vi "Logger2_Loop.vi"(8 "error in (no error)":errorcluster) -> (0 "error out":errorcluster)   [LabVIEW 2016]
uses:
  Classes/DataLogger/Data Logger.lvclass
  <vilib>/Platform/TimedLoop/XDataNode/timing_clust.ctl
  <vilib>/Platform/TimedLoop/XDataNode/nitl_modes.ctl
  <vilib>/Platform/TimedLoop/XDataNode/wakeup.ctl
  <vilib>/Platform/TimedLoop/XDataNode/XDataNode.xnode
  <vilib>/Platform/TimedLoop/XDataNode/XDNodeRunTimeDep.lvlib
  <vilib>/GoldZinc Software/auzn custom VIs/CustomVI.lvlib
panel:
  out "Save Time":dbl
  out "ColumnOfVar":i32[](array[numeric])
  out "NumOfColumn":i32
  out "StartTime":dbl
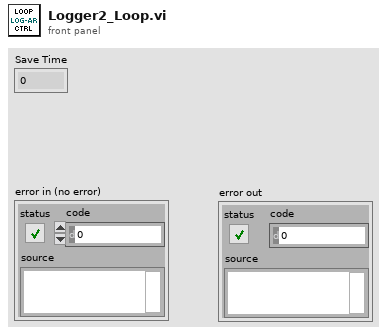
[diagram p1: front panel]
types:
  T1 = enum16{"Idle", "CloseFile", "WriteFile", "CreateFile"}
  T2 = typedef "XDNodeRunTimeDep.lvlib/timing_clust.ctl" = cluster{"Expected End [f-1]":u64, "Actual End [f-1]":u64, "Finished Late? [f-1]":bool, "Expected End [i-1]":u64, "Actual End [i-1]":u64, "Finished Late? [i-1]":bool, "Expected Start [i]":u64, "Actual Start [i]":u64, "Expected Start [f]":u64, "Actual Start [f]":u64, "Source Name":string, "Structure Name":string, "Period":i64, "Deadline":i64, "Offset":i64, "Start":i64, "Priority":i32, "Timeout":i32, "Mode":T3, "Wakeup Reason":T4, "Error":errorcluster, "Source Type":string, "Secondary Source Type":string, "Global End Time":u64, "Global Start Time":u64, "Frame Duration":u64, "Iteration Duration":u64, "Assigned CPU":i32, "I/O Scan Engine Mode":u32}
  T3 = typedef "XDNodeRunTimeDep.lvlib/nitl_modes.ctl" = enum32{"No Change", "Process missed periods, maintain original phase", "Discard missed periods, maintain original phase", "Process missed periods, ignore original phase", "Discard missed periods, ignore original phase"}
  T4 = typedef "XDNodeRunTimeDep.lvlib/wakeup.ctl" = enum32{"Normal", "Aborted", "Asynchronous wakeup", "Timing source error", "Timed loop error", "Timeout"}
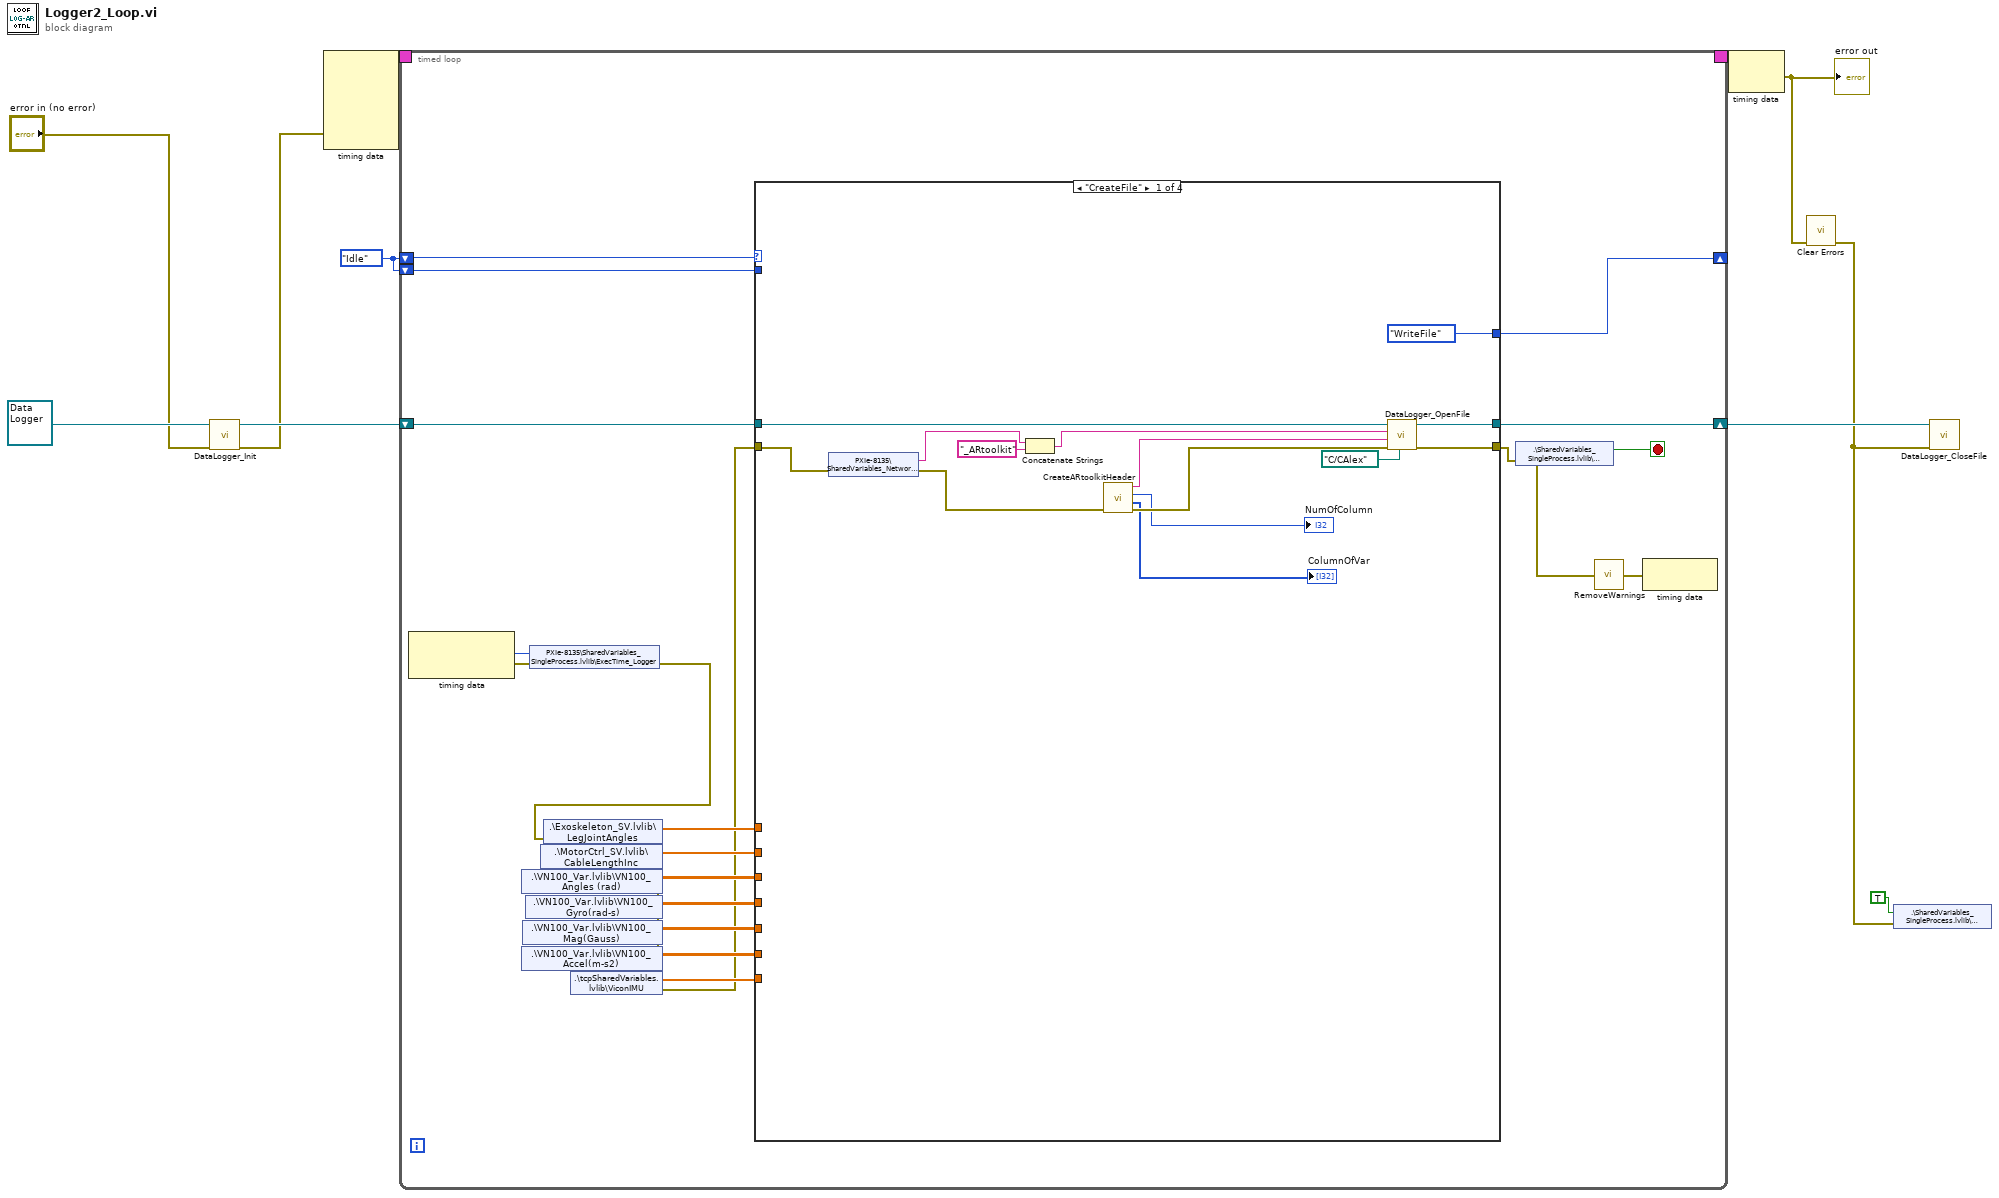
[diagram p0: block diagram]
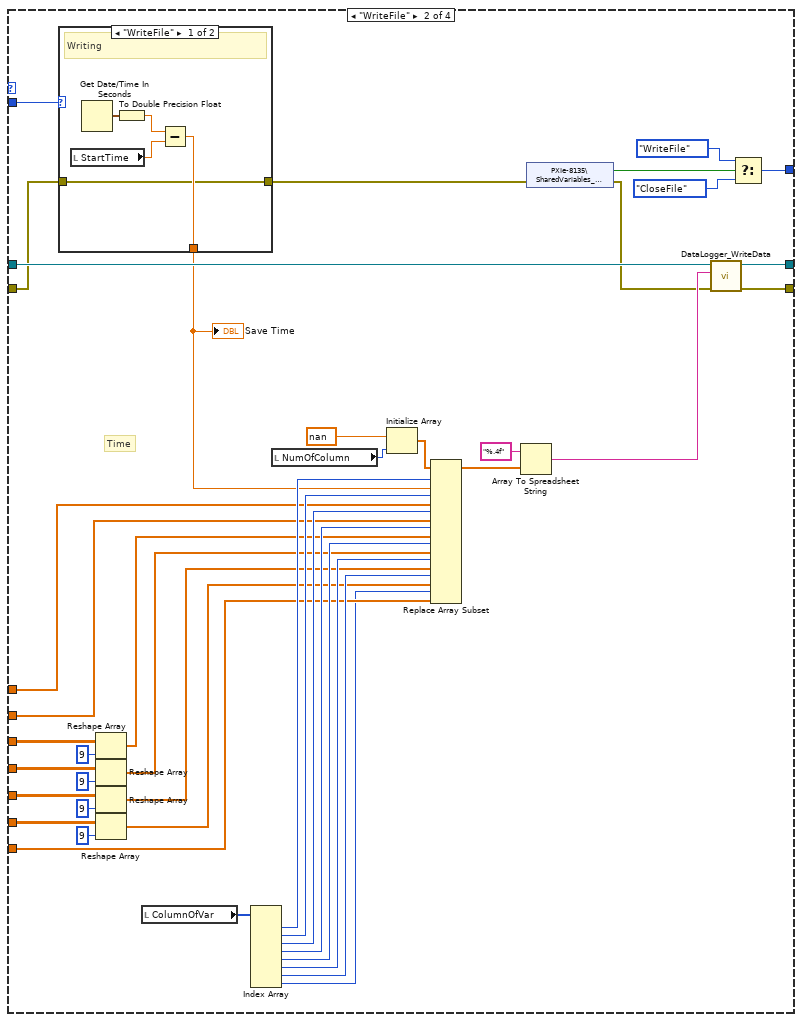
[diagram p2: hidden frame]
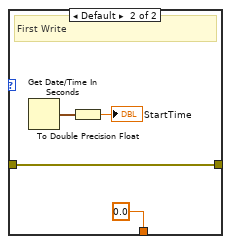
[diagram p3: hidden frame]
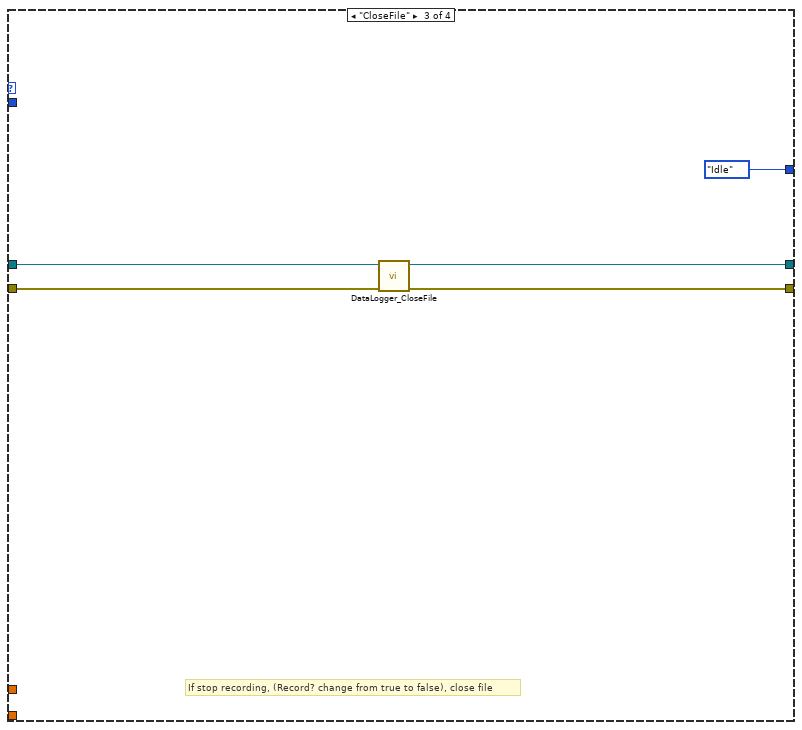
[diagram p4: hidden frame]
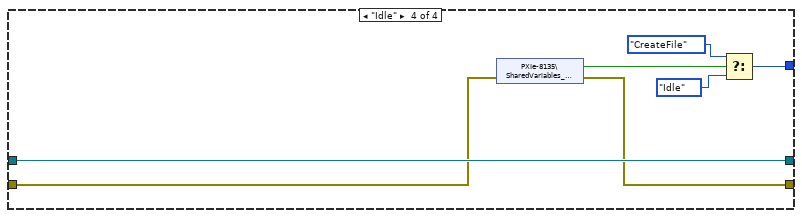
[diagram p5: hidden frame]
diagram:
  w9 = T1."Idle"
  n1 = call "DataLogger_Init.vi"("error in (no error)"="error in (no error)", "Data Logger in"=refnum<class "Data Logger.lvclass"> refnum) -> ("error out"=w1:errorcluster, "Data Logger out"=w3:refnum<class "Data Logger.lvclass">)  [unwired: 8 in]
  n2 = node-c288(w1) -> (w11:T2)  [unwired: 4 in]
  n3 = timed-loop {
    timing: w11 -> [_]
    timing-out: [_] -> w10
    shift-right: [w36] -> w7
    shift-left: w3 -> [w37]
    shift-right: [w35] -> _
    shift-left: w9 -> [w34]
    shift-left: w9 -> [w33]
    stop <- w31 stop-if-true
    n4 = node-c288() -> (w32:i64, w22:errorcluster)  [unwired: 1 in]
    n5 = shared-variable "PXIe-8135\\SharedVariables_SingleProcess.lvlib\\ExecTime_Logger"(w32, error in=w22) -> (error out=w17:errorcluster)
    n6 = shared-variable ".\\Exoskeleton_SV.lvlib\\LegJointAngles"(error in=w17) -> (w18:dbl[], error out=w15:errorcluster)
    n7 = shared-variable ".\\MotorCtrl_SV.lvlib\\CableLengthInc"(error in=w15) -> (w13:dbl[], error out=w14:errorcluster)
    n8 = shared-variable ".\\VN100_Var.lvlib\\VN100_Angles (rad)"(error in=w14) -> (w26:dbl[][], error out=w29:errorcluster)
    n9 = shared-variable ".\\VN100_Var.lvlib\\VN100_Gyro(rad-s)"(error in=w29) -> (w25:dbl[][], error out=w28:errorcluster)
    n10 = shared-variable ".\\VN100_Var.lvlib\\VN100_Mag(Gauss)"(error in=w28) -> (w24:dbl[][], error out=w27:errorcluster)
    n11 = shared-variable ".\\VN100_Var.lvlib\\VN100_Accel(m-s2)"(error in=w27) -> (w23:dbl[][], error out=w16:errorcluster)
    n12 = shared-variable ".\\tcpSharedVariables.lvlib\\ViconIMU"(error in=w16) -> (w19:dbl[], error out=w12:errorcluster)
    n13 = case shown="\"CreateFile\"" w34 {
      tunnel: w37 -> [w51 w89 w107 w114]
      tunnel: w12 -> [w50 w85 w103 w109]
      tunnel: [w48 w93 w105 w114] -> w36
      tunnel: [w42 w92 w104 w108] -> w30
      tunnel: [T1."WriteFile" w86 T1."Idle" w111] -> w35
      tunnel: w18 -> [_ w62 _ _]
      tunnel: w26 -> [_ w66 _ _]
      tunnel: w25 -> [_ w65 _ _]
      tunnel: w24 -> [_ w64 _ _]
      tunnel: w23 -> [_ w63 _ _]
      tunnel: w33 -> [_ w72 _ _]
      tunnel: w19 -> [_ w57 _ _]
      tunnel: w13 -> [_ w55 _ _]
      frame "CreateFile" {
        n14 = shared-variable "PXIe-8135\\SharedVariables_Network.lvlib\\FileName"(error in=w50) -> (w41:string, error out=w46:errorcluster)
        n15 = Concatenate Strings(w41, "_ARtoolkit" ("string")) -> (w40:string)
        n16 = call "CreateARtoolkitHeader.vi"("error in (no error)"=w46) -> ("error out"=w45:errorcluster, "Starting Column of Each Variable"=→"ColumnOfVar":i32[], "Number of Columns"=→"NumOfColumn":i32, "header"=w49:string)  [unwired: 7 in]
        n17 = call "DataLogger_OpenFile.vi"("base path (C:\\CAlex\\)"=path "C:/CAlex" ("base path (C:\\CAlex\\)"), "error in (no error)"=w45, "Header"=w49, "File Name"=w40, "Data Logger in"=w51) -> ("error out"=w42:errorcluster, "Data Logger out"=w48:refnum<class "Data Logger.lvclass">)  [unwired: 5 in]
      }
      frame "WriteFile" {
        # "Time"
        n18 = case shown="\"WriteFile\"" w72 {
          tunnel: w85 -> [w94 w99]
          tunnel: [w94 w99] -> w54
          tunnel: [w95 0.0 ("StartTime")] -> w71
          frame "WriteFile" {
            # "Writing"
            n19 = local read "StartTime"() -> (w96:dbl)
            n20 = Get Date/Time In Seconds() -> (seconds since 1Jan1904=w98:timestamp)
            n21 = To Double Precision Float(number=w98) -> (double precision float=w97:dbl)
            n22 = Subtract(x=w97, y=w96) -> (x-y=w95:dbl)
          }
          frame Default {
            # "First Write"
            n23 = Get Date/Time In Seconds() -> (seconds since 1Jan1904=w102:timestamp)
            n24 = To Double Precision Float(number=w102) -> (double precision float=→"StartTime":dbl)
          }
        }
        "Save Time" <- w71
        n25 = Reshape Array(w66, 9 ("dimension size")) -> (w61:dbl[])
        n26 = Reshape Array(w65, 9 ("dimension size")) -> (w60:dbl[])
        n27 = Reshape Array(w64, 9 ("dimension size")) -> (w59:dbl[])
        n28 = Reshape Array(w63, 9 ("dimension size")) -> (w58:dbl[])
        n29 = local read "ColumnOfVar"() -> (w80:i32[])
        n30 = Index Array(array=w80) -> (element #1=w79:i32, element #2=w78:i32, element #3=w77:i32, element #4=w76:i32, element #5=w75:i32, element #6=w74:i32, element #7=w73:i32, element #8=w56:i32)  [unwired: 8 in]
        n31 = local read "NumOfColumn"() -> (w81:i32)
        n32 = Initialize Array(nan ("element"), w81) -> (w91:dbl[])
        n33 = Replace Array Subset(array=w91, new element #1=w71, index #1=w79, new element #2=w62, index #2=w78, new element #3=w55, index #3=w77, new element #4=w61, index #4=w76, new element #5=w60, index #5=w75, new element #6=w59, index #6=w74, new element #7=w58, index #7=w73, new element #8=w57, index #8=w56) -> (w84:dbl[])
        n34 = Array To Spreadsheet String(array=w84, 3:"%.4f" ("format string")) -> (spreadsheet string=w83:string)  [unwired: 1 in]
        n35 = shared-variable "PXIe-8135\\SharedVariables_Network.lvlib\\Record?"(error in=w54) -> (w52:bool, error out=w53:errorcluster)
        n36 = call "DataLogger_WriteData.vi"("error in (no error)"=w53, "New line"=w83, "Data Logger in"=w89) -> ("error out"=w92:errorcluster, "Data Logger out"=w93:refnum<class "Data Logger.lvclass">)  [unwired: 7 in]
        n37 = Select(t=T1."WriteFile", s=w52, f=T1."CloseFile") -> (s? t:f=w86:T1)
      }
      frame "CloseFile" {
        # "If stop recording, (Record? change from true to false), close file"
        n38 = call "DataLogger_CloseFile.vi"("error in (no error)"=w103, "Data Logger in"=w107) -> ("error out"=w104:errorcluster, "Data Logger out"=w105:refnum<class "Data Logger.lvclass">)  [unwired: 8 in]
      }
      frame "Idle" {
        n39 = shared-variable "PXIe-8135\\SharedVariables_Network.lvlib\\Record?"(error in=w109) -> (w110:bool, error out=w108:errorcluster)
        n40 = Select(t=T1."CreateFile", s=w110, f=T1."Idle") -> (s? t:f=w111:T1)
      }
    }
    n41 = shared-variable ".\\SharedVariables_SingleProcess.lvlib\\GlobalStop"(error in=w30) -> (w31:bool, error out=w20:errorcluster)
    n42 = call <vilib>:"RemoveWarnings.vi"("error in (no error)"=w20) -> ("error out"=w21:errorcluster)
    n43 = node-c288(w21) -> ()  [unwired: 1 out]
  }
  n44 = node-c288(w10) -> (w6:errorcluster)
  "error out" <- w6
  n45 = call <vilib>:"Clear Errors.vi"("error in (no error)"=w6) -> ("error out"=w5:errorcluster)  [unwired: 5 in, 1 out]
  n46 = shared-variable ".\\SharedVariables_SingleProcess.lvlib\\GlobalStop"(TRUE ("GlobalStop"), error in=w5) -> ()  [unwired: 1 out]
  n47 = call "DataLogger_CloseFile.vi"("error in (no error)"=w5, "Data Logger in"=w7) -> ()  [unwired: 8 in, 2 out]
